vi "Throttle.vi"(10 "Throttle":dbl, 11 "Input":dbl) -> (3 "Output":dbl)   [LabVIEW 2017]
panel:
  in  "Base percent":dbl=0.5
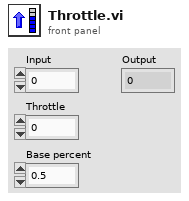
[diagram p1: front panel]
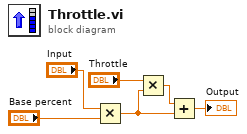
[diagram p0: block diagram]
diagram:
  n1 = Multiply(x="Input", y="Base percent") -> (x*y=w4:dbl)
  n2 = Multiply(x="Throttle", y=w4) -> (x*y=w6:dbl)
  n3 = Add(x=w6, y=w4) -> (x+y=→"Output":dbl)
